vi "SetReady.vi"(8 "error in (no error)":errorcluster, 10 "Ready":bool, 11 "reference in":refnum<class "DUT_Handler_Bailey_Panel.lvclass">) -> (0 "error out":errorcluster, 3 "reference in":refnum<class "DUT_Handler_Bailey_Panel.lvclass">)   [LabVIEW 2017]
uses:
  DUT_Handler_Bailey_Panel.lvclass
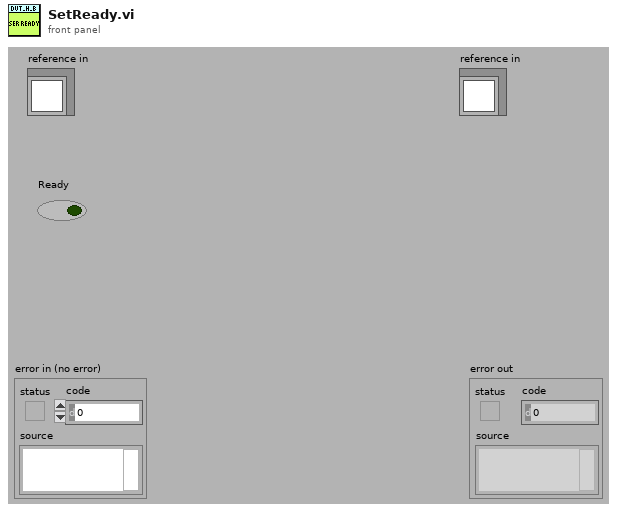
[diagram p1: front panel]
types:
  T1 = typedef "DUT_Handler_Bailey_Panel.lvlib/DUT_Handler_Bailey_Panel.lvclass/ObjectAttributes.ctl" = cluster{"Config":T2, "Barcode":refnum<class "Barcode_Reader_Base.lvclass">, "SN":string, "DUT":u32}
  T2 = typedef "DUT_Handler_Bailey_Panel.lvlib/DUT_Handler_Bailey_Panel.lvclass/Config.ctl" = cluster{"DUT Quantity":u32}
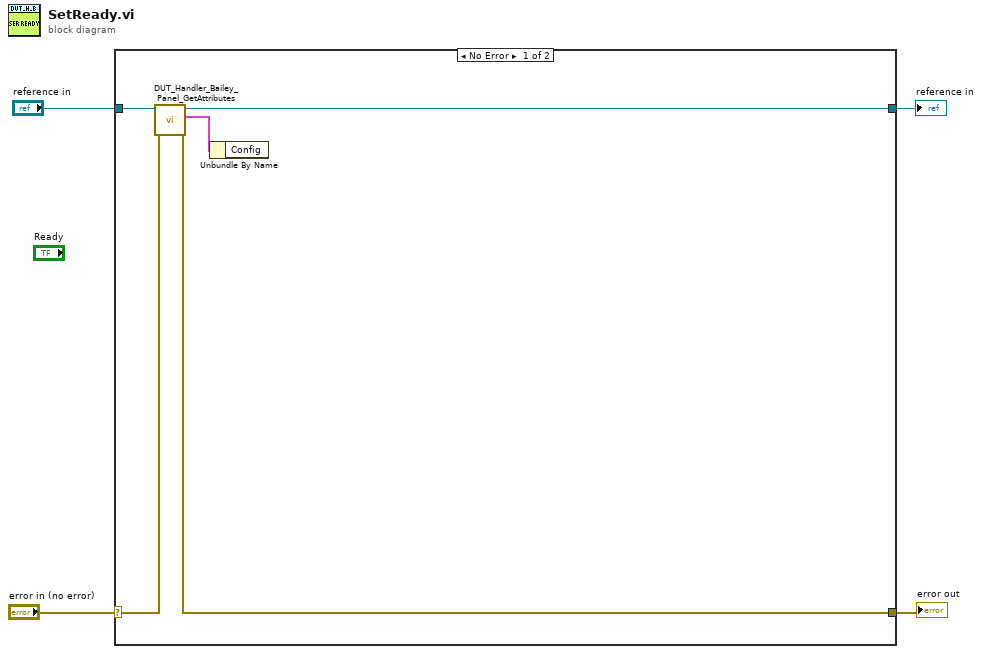
[diagram p0: block diagram]
diagram:
  n1 = case shown="No Error" "error in (no error)" {
    selector: "error in (no error)" -> [w9 w11]
    tunnel: [w7 w11] -> w3
    tunnel: [w5 w10] -> w1
    tunnel: "reference in" -> [w6 w10]
    frame No Error {
      n2 = call "DUT_Handler_Bailey_Panel_GetAttributes.vi"("error in (no error)"=w9, "reference in"=w6) -> ("error out"=w7:errorcluster, "Data"=w8:T1, "reference out"=w5:refnum<class "DUT_Handler_Bailey_Panel.lvclass">)  [unwired: 6 in, 1 out]
      n3 = Unbundle By Name(w8) -> ()  [unwired: 1 out]
    }
    frame Error {
    }
  }
  "error out" <- w3
  "reference in" <- w1
